vi "DP I-O (F1L1).vi"(11 "Expt State (in)":T4) -> (3 "State":T4)   [LabVIEW 2020]
uses:
  Typedefs/DP-Stim Params (F1L1).ctl
  epl-vi-lib/Utility VIs/Type Defs/Left-Right ring.ctl
  CFTS Main Panel SubVIs/CFTS-Experiment State.ctl
  Typedefs/DP-StimGen.ctl
  Typedefs/DP-Rejection Settings.ctl
  CFTS Main Panel SubVIs/CFTS-Data Type Enum.ctl
panel:
  out "exit signal":bool
  in  "Reject":T1 caption="Rejection"
  in  "StimGen":T2={"Sampling Rate (Hz)"=200000.0, "Npts"=10000, "Data Folder"=path "", "Acoustic System"="", "Recalibrate?"=FALSE, "AO Channels"=[], "Mic  gain (dB)"=0.0, "F1, F2 speakers"=[], "Override recal check"=FALSE}
  out "Freqs":cluster{"f1":dbl, "f2":dbl, "2f1-f2":dbl}={"f1"=9419.759114583332, "f2"=11291.50390625, "2f1-f2"=7548.014322916664} {"2f1-f2" format="%.3f"; "f1" format="%.3f"; "f2" format="%.3f"}
  out "Abort":bool
  in  "Recalibrate":bool
  in  "Probe Mic Gain (dB)":dbl
  in  "Save Waves?":bool=TRUE
  out "User":string
  out "Run #":u16=14
  out "ID #":u16=1
  in  "Avg specs":T3={"# Time avgs "=8, "# Spectrum avgs"=4}
  out "running":bool
  out "Path":path
  in  "DP Params":T5={"Start (dB)"=20.0, "Stop (dB)"=70.0, "Step (dB)"=10.0, "Ear"=enum."Right", "f2 (kHz)"="5.6;8.0;11.3;16;22.6;32;", "f1"=1.2, "f1 mode"=enum."re f2", "L1"=10.0, "L1 mode"=enum."re L2"}
  out "DP window":cluster{i32, "df (Hz)":dbl, dbl[]}(graph)={0, "df (Hz)"=0.02, []}
  out "I-O Plot":cluster{cluster{dbl, dbl}[]}[](graph)
  in  "Notes":string
  out "Full Spectrum":cluster{i32, "Freq Resolution":dbl, dbl[]}(graph)={0, "Freq Resolution"=20.345052083333332, []}
  in  "RETURN":bool
  in  "START":bool
  in  "STOP":bool
  # "Stimulus"
  # "Averaging"
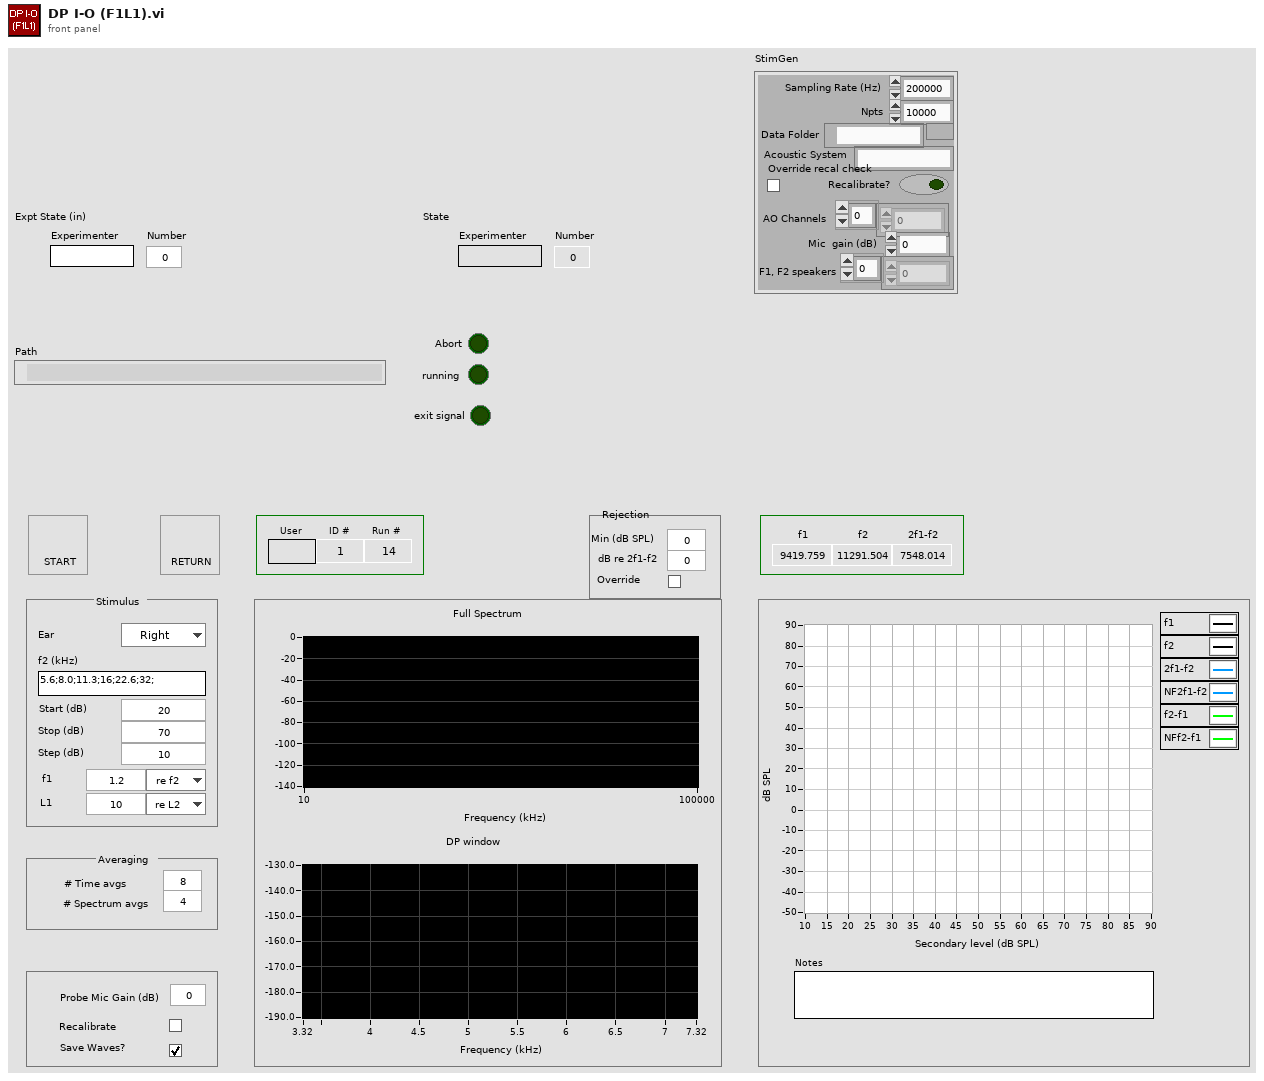
[diagram p1: front panel]
types:
  T1 = typedef "DP-Rejection Settings.ctl" = cluster{"Override":bool, "dB re 2f1-f2":dbl, "Min (dB SPL)":dbl}
  T2 = typedef "DP-StimGen.ctl" = cluster{"Sampling Rate (Hz)":dbl, "Npts":i32, "Data Folder":path, "Acoustic System":string, "Recalibrate?":bool, "AO Channels":i32[], "Mic  gain (dB)":dbl, "F1, F2 speakers":i32[], "Override recal check":bool}
  T3 = cluster{"# Time avgs ":i32, "# Spectrum avgs":i32}
  T4 = typedef "CFTS-Experiment State.ctl" = cluster{"Experimenter":string, "Number":u32, "Right":string, "Left":string, "Data Folder":path, "State File":path, "Version Info":string, "End Exposure Time":dbl, "Exposure Duration":string, "Run #":cluster{"CAP":i16, "ABR":i16, "DP":i16, "VsEP":i16, "MeasSeq":i16, "SubSeq":i16, "SFOAE":i16}}
  T5 = typedef "DP-Stim Params (F1L1).ctl" = cluster{"Start (dB)":dbl, "Stop (dB)":dbl, "Step (dB)":dbl, "Ear":T6, "f2 (kHz)":string, "f1":dbl, "f1 mode":enum16{"re f2", "kHz"}, "L1":dbl, "L1 mode":enum16{"re L2", "dB"}}
  T6 = typedef "Left-Right ring.ctl" = enum16{"Right", "Left"}
  T7 = typedef "CFTS-Data Type Enum.ctl" = enum16{"CAP", "ABR", "DP", "VsEP", "MeasSeq", "SFOAE"}
  T8 = typedef "DP-Freqs.ctl" = cluster{"f1":dbl, "f2":dbl, "2f1-f2":dbl}
  T9 = typedef "DP-DataAcq.ctl" = cluster{"#spectra avgs":i32[], "#time avgs":i32[], "dt (ms)":dbl, "df (kHz)":dbl, "Npts":i32, "Save waves?":bool, "Data File":path, "AI Channels":u16[], "Sampling rate (Hz)":dbl, "Probe Tube Sensitivity":cluster{"Frequency":dbl[], "Mag":dbl[]}, "Mic gain (dB)":dbl, "ptIndex":i32}
  T10 = typedef "CFTS-Options.ctl" = cluster{"DP Artifact Rejection":bool, "Monitor vital signs ":bool, "Extension":string}
  T11 = cluster{"Shift":bool, "Ctrl":bool, "Alt":bool, "Cmd":bool, "Opt":bool}
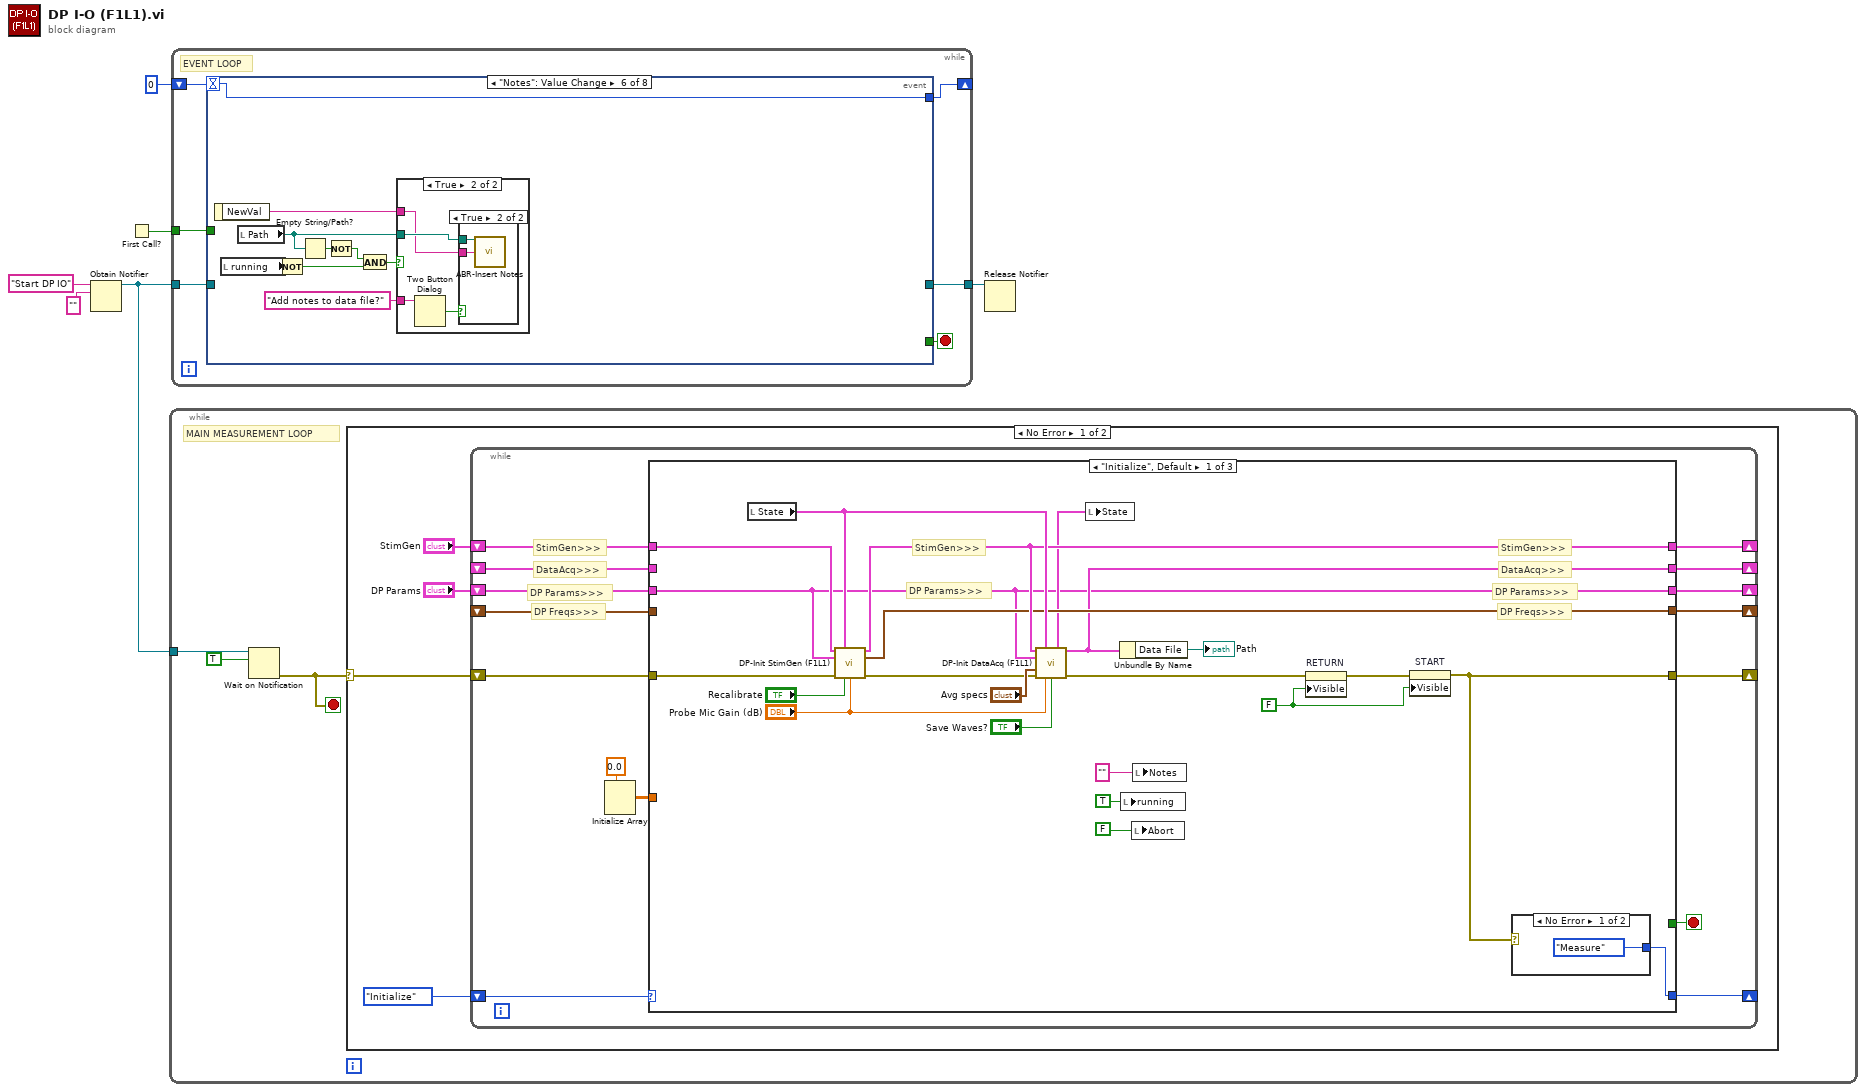
[diagram p0: block diagram]
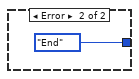
[diagram p2: hidden frame]
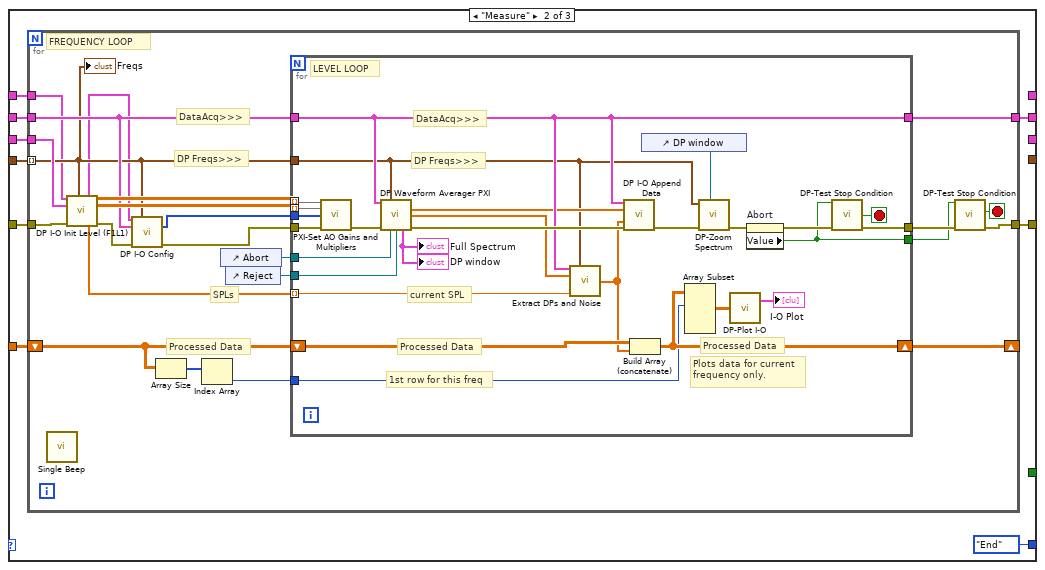
[diagram p3: hidden frame]
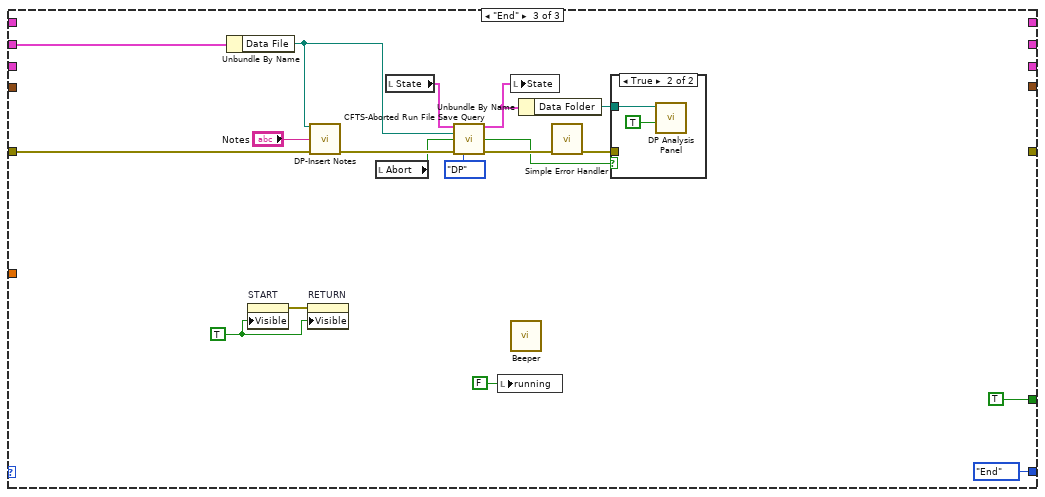
[diagram p4: hidden frame]
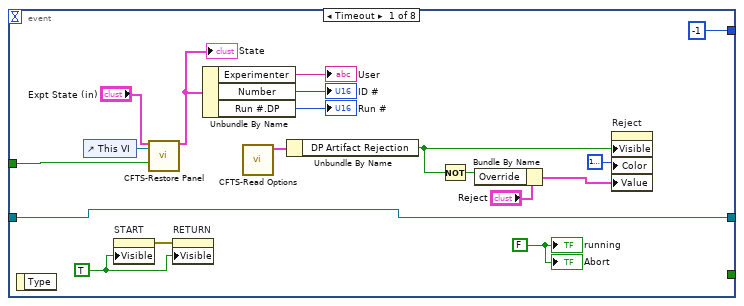
[diagram p7: hidden frame]
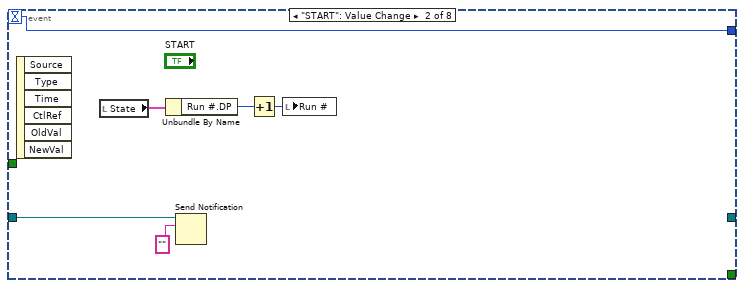
[diagram p8: hidden frame]
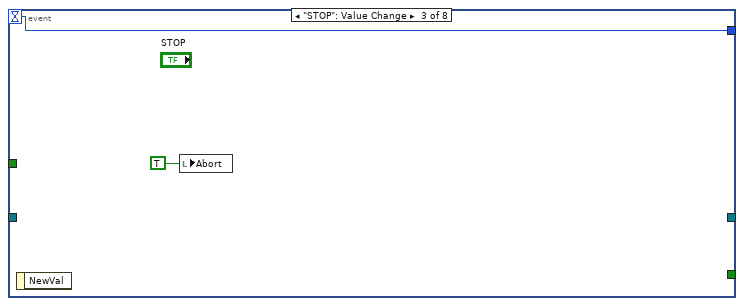
[diagram p9: hidden frame]
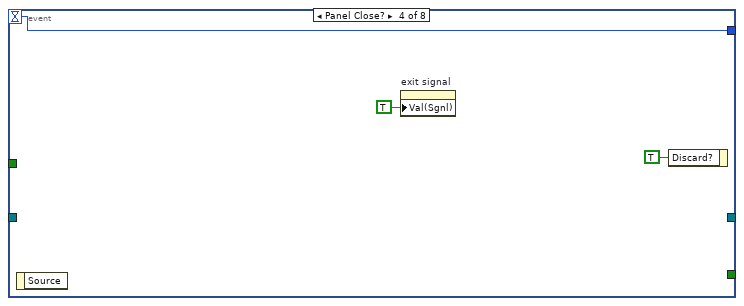
[diagram p10: hidden frame]
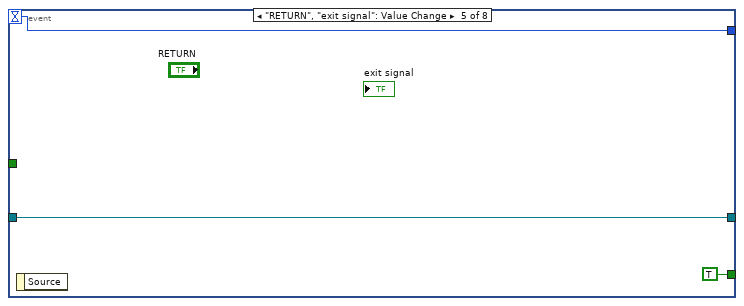
[diagram p11: hidden frame]
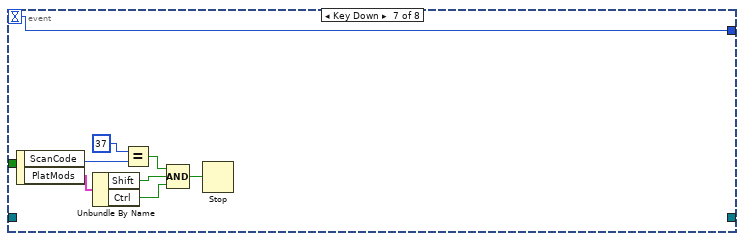
[diagram p14: hidden frame]
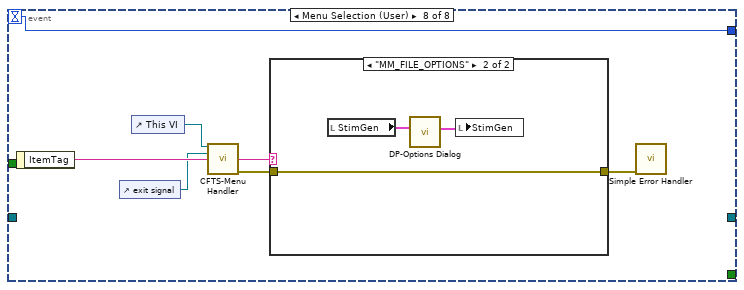
[diagram p15: hidden frame]
diagram:
  n1 = Obtain Notifier(name (unnamed)="Start DP IO", notification data type="") -> (notifier out=w6:refnum<notifier>)  [unwired: 2 in, 2 out]
  n2 = First Call?() -> (First Call?: T/F=w1:bool)
  n3 = while {
    tunnel: w6 -> [w8]
    stop <- w7 stop-if-true
    # "MAIN MEASUREMENT LOOP"
    n4 = Wait on Notification(notifier=w8, ignore previous (F)=TRUE) -> (error out=w7:errorcluster)  [unwired: 2 in, 3 out]
    n5 = case shown="No Error" w7 {
      selector: w7 -> [w10 _]
      frame No Error {
        n6 = while {
          shift-right: [w27] -> _
          shift-left: w10 -> [w28]
          shift-right: [w18] -> _
          shift-left: enum16{"Initialize", "Measure", "End"}."Initialize" -> [w26]
          shift-right: [w22] -> _
          shift-left: "StimGen" -> [w24]
          shift-right: [w21] -> _
          shift-left: _ -> [w23]
          shift-right: [w19] -> _
          shift-left: "DP Params" -> [w20]
          shift-right: [w17] -> _
          shift-left: _ -> [w16]
          stop <- w25 stop-if-true
          # "DP Freqs>>>"
          # "DP Params>>>"
          # "DataAcq>>>"
          # "StimGen>>>"
          n7 = Initialize Array(0.0) -> (w14:dbl[][])  [unwired: 2 in]
          n8 = case shown="\"Initialize\", Default" w26 {
            tunnel: w28 -> [w41 w61 w121]
            tunnel: [w31 w60 _] -> w27
            tunnel: [_ _ TRUE] -> w25
            tunnel: w24 -> [w43 w57 _]
            tunnel: w23 -> [_ w55 w122]
            tunnel: [w42 _ _] -> w22
            tunnel: [w33 w53 _] -> w21
            tunnel: w20 -> [w29 w56 _]
            tunnel: [w29 _ _] -> w19
            tunnel: [w30 enum16{"Initialize", "Measure", "End"}."End" enum16{"Initialize", "Measure", "End"}."End"] -> w18
            tunnel: [w36 _ _] -> w17
            tunnel: w16 -> [_ w58 _]
            tunnel: w14 -> [_ w59 _]
            frame "Initialize", Default {
              w47 = FALSE
              # "DP Freqs>>>"
              # "DP Params>>>"
              # "StimGen>>>"
              # "DP Params>>>"
              # "DataAcq>>>"
              # "StimGen>>>"
              n9 = local read "State"() -> (w44:T4)
              n10 = call "DP-Init StimGen (F1L1).vi"("StimGen"=w43, "Expt State"=w44, "DP stimulus params"=w29, "error in (no error)"=w41, "Recalibrate?"="Recalibrate", "Mic  gain (dB)"="Probe Mic Gain (dB)") -> ("StimGen (out)"=w42:T2, "DP Freqs"=w36:T8[], "error out"=w40:errorcluster)  [unwired: 7 in]
              n11 = call "DP-Init DataAcq (F1L1).vi"("StimGen"=w42, "Expt State"=w44, "DP stimulus params"=w29, "Avg specs"="Avg specs", "error in (no error)"=w40, "Mic gain (dB)"="Probe Mic Gain (dB)", "Save waves?"="Save Waves?") -> ("Expt State out"=w34:T4, "DataAcq"=w33:T9, "error out"=w38:errorcluster)  [unwired: 6 in]
              n12 = local write "State"(w34) -> ()
              n13 = Unbundle By Name(w33) -> ("Data File"=→"Path":path)
              n14 = local write "running"(TRUE ("running")) -> ()
              n15 = local write "Abort"(FALSE ("Stopping")) -> ()
              n16 = local write "Notes"("" ("Notes")) -> ()
              n17 = property on="RETURN" class="Bool"(error in=w38, "Visible"=w47) -> (error out=w37:errorcluster)  [unwired: 1 in, 1 out]
              n18 = property on="START" class="Bool"(error in=w37, "Visible"=w47) -> (error out=w31:errorcluster)  [unwired: 1 in, 1 out]
              n19 = case shown="No Error" w31 {
                tunnel: [enum16{"Initialize", "Measure", "End"}."Measure" enum16{"Initialize", "Measure", "End"}."End"] -> w30
                frame No Error {
                }
                frame Error {
                }
              }
            }
            frame "Measure" {
              n20 = for {
                shift-right: [w75] -> _
                shift-left: w59 -> [w82]
                tunnel: w61 -> [w79]
                tunnel: [w67] -> w60
                tunnel: w58 -> [w71] mode=indexing
                tunnel: w57 -> [w63]
                tunnel: w56 -> [w74]
                tunnel: w55 -> [w72]
                tunnel: [w70] -> w53
                stop <- w73 stop-if-true
                # "DP Freqs>>>"
                # "DataAcq>>>"
                # "FREQUENCY LOOP"
                # "Processed Data"
                # "SPLs"
                n21 = call "Single Beep.vi"() -> ()  [unwired: 1 in]
                n22 = call "DP I-O Init Level (F1L1).vi"("StimGen"=w63, "DP Freqs"=w71, "DP stimulus params"=w74, "error in (no error)"=w79) -> ("StimGen Out"=w62:T2, "Multipliers (2D)"=w84:dbl[][], "Gains (2D)"=w83:dbl[][], "Nominal f2 SPL"=w76:dbl[], "error out"=w78:errorcluster)  [unwired: 7 in]
                n23 = call "DP I-O Config.vi"("StimGen"=w62, "DP Freqs"=w71, "DataAcq"=w72, "error in (no error)"=w78) -> ("AO Channels"=w69:i32[], "error out"=w77:errorcluster)  [unwired: 10 in]
                n24 = Array Size(array=w82) -> (size(s)=w81:i32[])
                n25 = Index Array(array=w81) -> (element=w80:i32)  [unwired: 1 in]
                n26 = control-ref of="Abort"() -> (w65:refnum<vi>)
                n27 = control-ref of="Reject"() -> (w64:refnum<vi>)
                n28 = for {
                  tunnel: w84 -> [w110] mode=indexing
                  tunnel: w83 -> [w109] mode=indexing
                  tunnel: w76 -> [w96] mode=indexing
                  shift-right: [w106] -> w75
                  shift-left: w82 -> [w108]
                  tunnel: w80 -> [w104]
                  tunnel: w77 -> [w111]
                  tunnel: [w91] -> w68
                  tunnel: w72 -> [w95]
                  tunnel: w71 -> [w87]
                  tunnel: [w95] -> w70
                  tunnel: w69 -> [w92]
                  tunnel: [w88] -> w66
                  tunnel: w65 -> [w86]
                  tunnel: w64 -> [w85]
                  stop <- w102 stop-if-true
                  # "DP Freqs>>>"
                  # "DataAcq>>>"
                  # "LEVEL LOOP"
                  # "current SPL"
                  # "Plots data for current\nfrequency only."
                  # "1st row for this freq"
                  # "Processed Data"
                  # "Processed Data"
                  n29 = call "PXI-Set AO Gains and Multipliers.vi"("Multipliers"=w110, "Gains"=w109, "AO Channels"=w92, "error in (no error)"=w111) -> ("error out"=w101:errorcluster)  [unwired: 11 in]
                  n30 = call "DP Waveform Averager PXI.vi"("DataAcq"=w95, "DP Freqs"=w87, "error in"=w101, "Abort"=w86, "Reject Ref"=w85) -> ("Ave Wave"=w94:dbl[], "Averaged Spectrum (Vrms)"=w98:dbl[], "waveform cluster"=→"Full Spectrum" →"DP window":cluster{i32, "dx":dbl, "Array":dbl[]}, "error out"=w100:errorcluster)  [unwired: 5 in, 2 out]
                  n31 = call "Extract DPs and Noise.vi"("DataAcq"=w95, "DP Freqs"=w87, "Spectrum in Vrms"=w98, "SPL"=w96) -> ("Output Array"=w97:dbl[])  [unwired: 11 in]
                  n32 = call "DP I-O Append Data.vi"("DataAcq"=w95, "Waveform"=w94, "Processed data"=w97, "error in (no error)"=w100) -> ("error out"=w103:errorcluster)  [unwired: 11 in]
                  n33 = Build Array (concatenate)(w108, w97) -> (w106:dbl[][])
                  n34 = control-ref of="DP window"() -> (w93:refnum<vi>)
                  n35 = Array Subset(array=w106, index (row)=w104) -> (w105:dbl[][])  [unwired: 3 in]
                  n36 = call "DP-Zoom Spectrum.vi"("DP window"=w93, "error in (no error)"=w103, "DP Freqs"=w87) -> ("error out"=w90:errorcluster)  [unwired: 8 in]
                  n37 = call "DP-Plot I-O.vi"("Input Array (4xn)"=w105) -> ("Current I-O Plot"=→"I-O Plot":cluster{cluster{dbl, dbl}[]}[])  [unwired: 1 out]
                  n38 = property on="Abort" class="Bool (strict)"(error in=w90) -> (error out=w89:errorcluster, "Value"=w88:bool)  [unwired: 1 in, 1 out]
                  n39 = call "DP-Test Stop Condition.vi"("Abort?"=w88, "error in (no error)"=w89) -> ("Stop?"=w102:bool, "error out"=w91:errorcluster)  [unwired: 12 in]
                }
                n40 = call "DP-Test Stop Condition.vi"("Abort?"=w66, "error in (no error)"=w68) -> ("Stop?"=w73:bool, "error out"=w67:errorcluster)  [unwired: 12 in]
                "Freqs" <- w71
              }
            }
            frame "End" {
              w128 = TRUE
              n41 = Unbundle By Name(w122) -> ("Data File"=w118:path)
              n42 = property on="START" class="Bool"("Visible"=w128) -> (error out=w124:errorcluster)  [unwired: 2 in, 1 out]
              n43 = property on="RETURN" class="Bool"(error in=w124, "Visible"=w128) -> ()  [unwired: 1 in, 2 out]
              n44 = call "DP-Insert Notes.vi"("path"=w118, "Notes"="Notes", "error in (no error)"=w121) -> ("error out"=w123:errorcluster)  [unwired: 12 in]
              n45 = local read "Abort"() -> (w116:bool)
              n46 = local read "State"() -> (w119:T4)
              n47 = call "CFTS-Aborted Run File Save Query.vi"("Expt State"=w119, "Path"=w118, "Aborted"=w116, "error in (no error)"=w123, "Data Type"=CFTS-Data_Type_Enum."DP") -> ("Expt State out"=w115:T4, "File saved?"=w113:bool, "error out"=w120:errorcluster)  [unwired: 8 in]
              n48 = local write "running"(FALSE ("running")) -> ()
              n49 = local write "State"(w115) -> ()
              n50 = call "Beeper.vi"() -> ()  [unwired: 5 in, 1 out]
              n51 = Unbundle By Name(w115) -> ("Data Folder"=w114:path)
              n52 = call <vilib>:"Simple Error Handler.vi"("error in (no error)"=w120) -> ("error out"=w112:errorcluster)  [unwired: 4 in, 4 out]
              n53 = case shown="True" w113 {
                tunnel: w114 -> [_ w131]
                tunnel: w112 -> [_ _]
                frame False {
                }
                frame True {
                  n54 = call "DP Analysis Panel.vi"("Autosave? (F)"=TRUE, "Data folder in"=w131) -> ()  [unwired: 10 in]
                }
              }
            }
          }
        }
      }
      frame Error {
      }
    }
  }
  n55 = while {
    tunnel: w6 -> [w137]
    shift-right: [w134] -> _
    shift-left: 0 -> [w135]
    tunnel: [w133] -> w2
    tunnel: w1 -> [w132]
    stop <- w136 stop-if-true
    # "EVENT LOOP"
    n56 = event shown="[5] \"Notes\": Value Change" {
      selector: _ -> [_ _ _ _ _ _ _ _]
      dyn-events: _ -> [_ _ _ _ _ _ _ _]
      timeout: w135 -> [_ w156 w163 w165 w168 w170 w192 w199]
      tunnel: w137 -> [w148 w161 _ _ w167 _ _ _]
      tunnel: [_ _ _ _ TRUE _ _ _] -> w136
      tunnel: [-1 w156 w163 w165 w168 w170 w192 w199] -> w134
      tunnel: [w148 _ _ _ w167 _ _ _] -> w133
      tunnel: w132 -> [w147 _ _ _ _ _ _ _]
      event Timeout {
        w151 = TRUE
        w150 = FALSE ("quitting")
        n57 = event-data() -> ()  [unwired: 1 in, 1 out]
        n58 = control-ref of="This VI"() -> (w146:refnum<vi>)
        n59 = property on="START" class="Bool"("Visible"=w151) -> (error out=w149:errorcluster)  [unwired: 2 in, 1 out]
        n60 = call "CFTS-Restore Panel.vi"("State (in)"="Expt State (in)", "VI refnum"=w146, "Restore?"=w147) -> ("State"=w144:T4)  [unwired: 11 in, 1 out]
        "State" <- w144
        n61 = property on="RETURN" class="Bool"(error in=w149, "Visible"=w151) -> ()  [unwired: 1 in, 2 out]
        n62 = Unbundle By Name(w144) -> ("Experimenter"=→"User":string, "Number"=→"ID #":u32, "Run #.DP"=→"Run #":i16)
        n63 = call "CFTS-Read Options.vi"() -> ("CFTS Options"=w143:T10)  [unwired: 10 in, 1 out]
        n64 = Unbundle By Name(w143) -> ("DP Artifact Rejection"=w139:bool)
        n65 = Not(x=w139) -> (.not. x?=w140:bool)
        n66 = Bundle By Name(cluster="Reject", "Override"=w140) -> (w138:T1)
        n67 = property on="Reject" class="Clust (strict)"("Visible"=w139, "Color"=u32 16777238, "Value"=w138) -> ()  [unwired: 2 in, 2 out]
        "running" <- w150
        "Abort" <- w150
      }
      event "START": Value Change {
        n68 = event-data() -> ()  [unwired: 1 in, 6 out]
        n69 = local read "State"() -> (w158:T4)
        n70 = Unbundle By Name(w158) -> ("Run #.DP"=w157:i16)
        n71 = Send Notification(notification="", notifier=w161) -> ()  [unwired: 1 in, 2 out]
        n72 = Increment(x=w157) -> (x+1=w159:i16)
        n73 = local write "Run #"(w159) -> ()
      }
      event "STOP": Value Change {
        n74 = event-data() -> ()  [unwired: 1 in, 1 out]
        n75 = local write "Abort"(TRUE ("Stopping")) -> ()
      }
      event Panel Close? {
        n76 = event-data() -> ()  [unwired: 1 in, 1 out]
        n77 = property on="exit signal" class="Bool (strict)"("Val(Sgnl)"=TRUE ("Value (Signaling)")) -> ()  [unwired: 2 in, 2 out]
        n78 = event-data("Discard?"=TRUE) -> ()  [unwired: 1 in, 1 out]
      }
      event "RETURN", "exit signal": Value Change {
        n79 = event-data() -> ()  [unwired: 1 in, 1 out]
      }
      event "Notes": Value Change {
        n80 = event-data() -> ("NewVal"=w173:string)  [unwired: 1 in]
        n81 = local read "running"() -> (w171:bool)
        n82 = local read "Path"() -> (w172:path)
        n83 = Not(x=w171) -> (.not. x?=w175:bool)
        n84 = Empty String/Path?(string/path=w172) -> (empty?=w174:bool)
        n85 = Not(x=w174) -> (.not. x?=w176:bool)
        n86 = And(x=w176, y=w175) -> (x .and. y?=w177:bool)
        n87 = case shown="True" w177 {
          tunnel: w172 -> [_ w182]
          tunnel: w173 -> [_ w181]
          tunnel: "Add notes to data file?" ("message") -> [_ w180]
          frame False {
          }
          frame True {
            n88 = Two Button Dialog(message=w180) -> (T button?=w179:bool)  [unwired: 2 in]
            n89 = case shown="True" w179 {
              tunnel: w182 -> [_ w184]
              tunnel: w181 -> [_ w183]
              frame False {
              }
              frame True {
                n90 = call "ABR-Insert Notes.vi"("path"=w184, "Notes"=w183) -> ()  [unwired: 12 in, 2 out]
              }
            }
          }
        }
      }
      event Key Down {
        n91 = event-data() -> ("ScanCode"=w191:i16, "PlatMods"=w189:T11)  [unwired: 1 in]
        n92 = Unbundle By Name(w189) -> ("Shift"=w187:bool, "Ctrl"=w186:bool)
        n93 = Equal?(x=i16 37 ("y"), y=w191) -> (x = y?=w188:bool)
        n94 = Compound Arithmetic op=AND(w188, w187, w186) -> (w185:bool)
        n95 = Stop(stop? (T)=w185) -> ()
      }
      event Menu Selection (User) {
        n96 = event-data() -> ("ItemTag"=w197:string)  [unwired: 1 in]
        n97 = control-ref of="exit signal"() -> (w193:refnum<vi>)
        n98 = control-ref of="This VI"() -> (w198:refnum<vi>)
        n99 = call "CFTS-Menu Handler.vi"("VI Refnum"=w198, "Return Refnum"=w193, "ItemTag"=w197) -> ("ItemTag out"=w196:string, "error out"=w195:errorcluster)  [unwired: 11 in]
        n100 = case shown="\"MM_FILE_OPTIONS\"" w196 {
          tunnel: w195 -> [w200 w203]
          tunnel: [w200 w203] -> w194
          frame "False", Default {
          }
          frame "MM_FILE_OPTIONS" {
            n101 = local read "StimGen"() -> (w202:T2)
            n102 = call "DP-Options Dialog.vi"("StimGen"=w202) -> ("StimGen out"=w201:T2)  [unwired: 8 in, 2 out]
            n103 = local write "StimGen"(w201) -> ()
          }
        }
        n104 = call <vilib>:"Simple Error Handler.vi"("error in (no error)"=w194) -> ()  [unwired: 4 in, 5 out]
      }
    }
  }
  n105 = Release Notifier(notifier=w2) -> ()  [unwired: 2 in, 3 out]
